vi "ThermoV_ControlSweep_2VO_VG2_nomean_160921.vi"() -> ()   [LabVIEW 2013]
panel:
  out "time/(60*13) indicator":dbl
  out "VGate Mod10 indicator":dbl
  in  "Operate HVpp\nOutput Timer":bool caption="Reset"
  out "modular 13":dbl
  in  "Number of seconds for \neach HVpp case state":dbl=30.0
  out "Elapsed Time (s)":dbl
  out "DC Value":dbl[](array[numeric]) format="%#.6f"
  in  "Saving Avg?":bool
  in  "Filename":path=path "trial_1.lvm"
  in  "STOP":bool
  in  "Save Waveform":bool
  out "Peak2Peak V":dbl[](array[numeric])
  out "Waveform Chart":dynamicdata(graph)
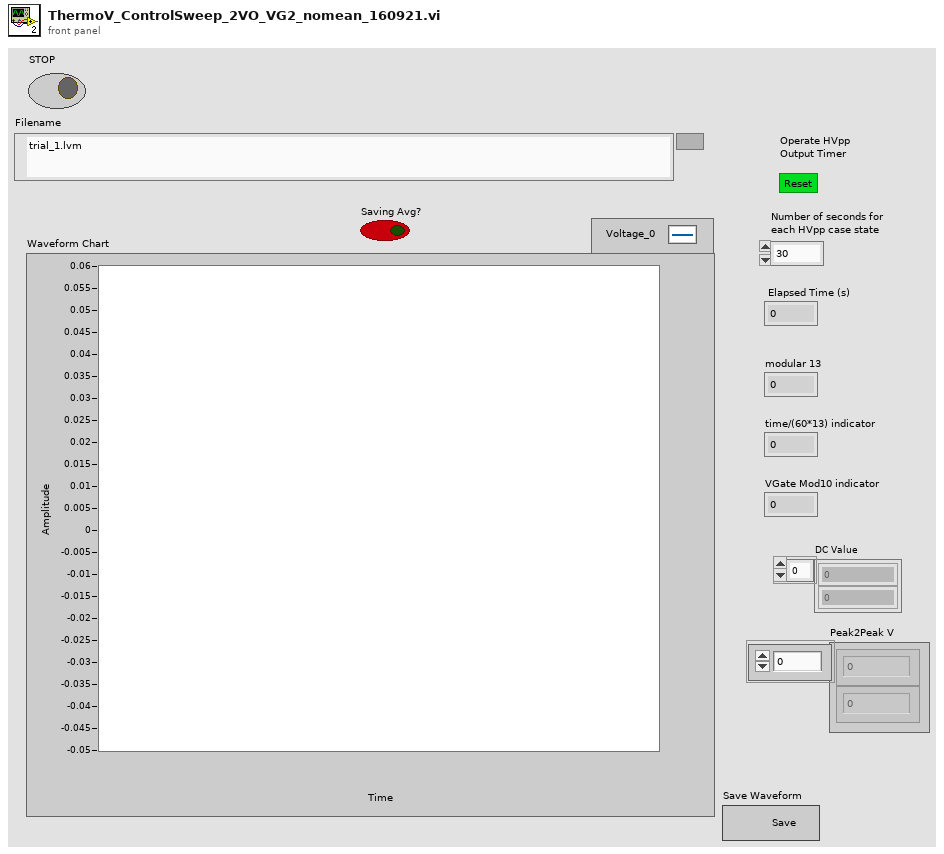
[diagram p1: front panel]
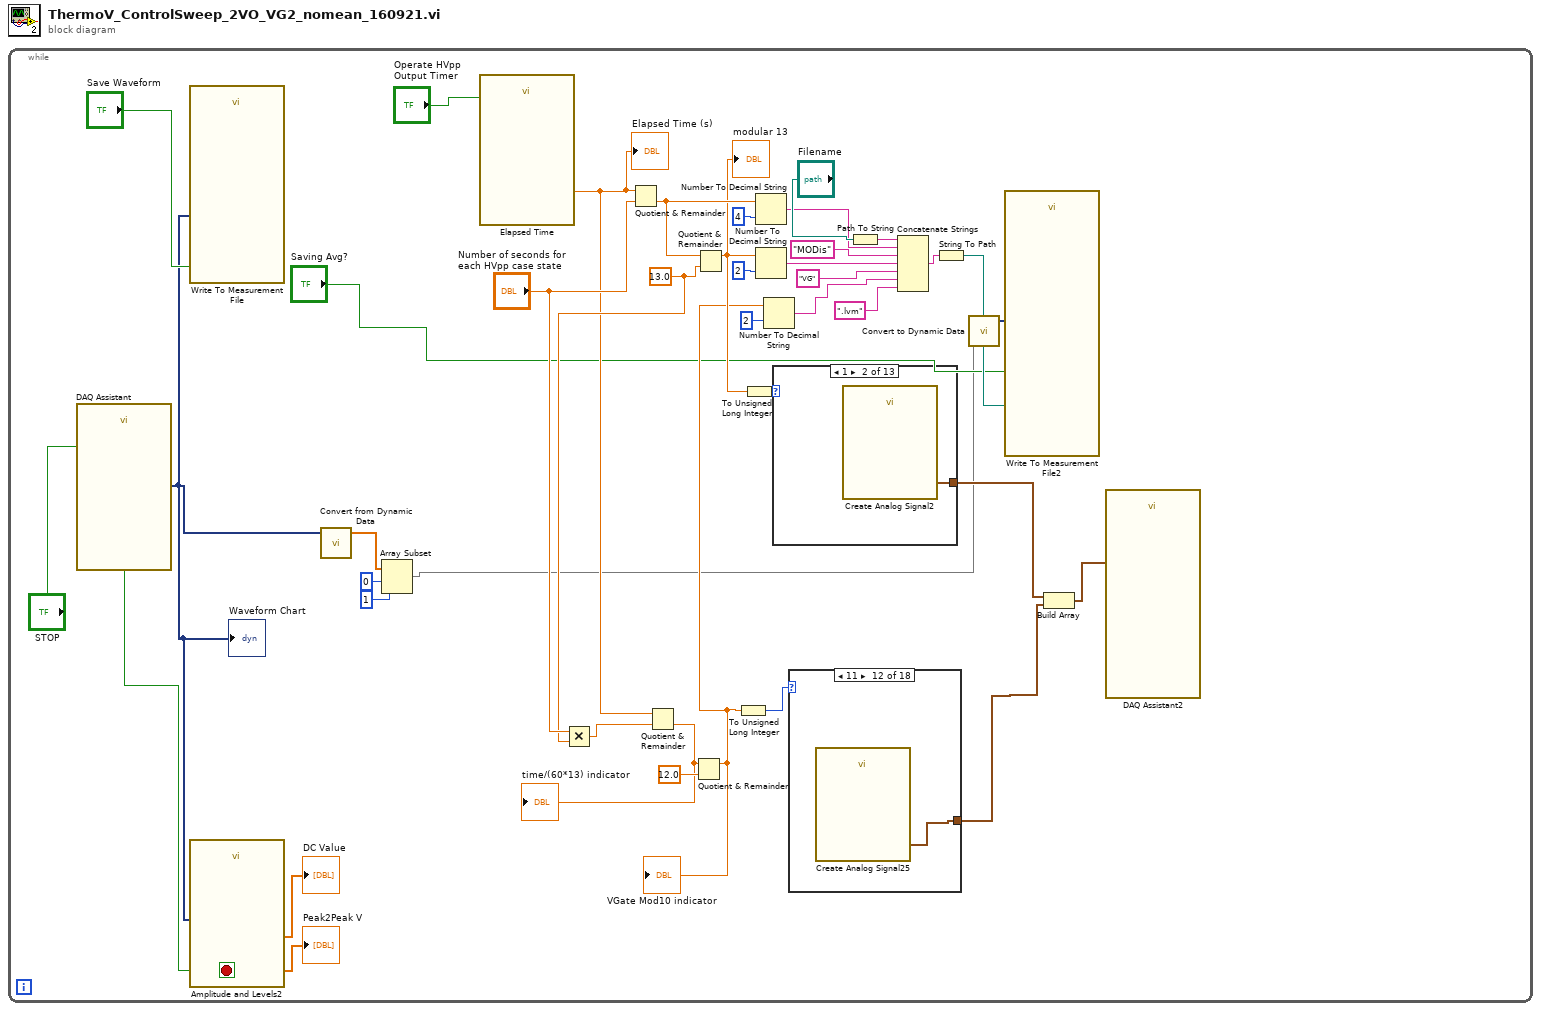
[diagram p0: block diagram]
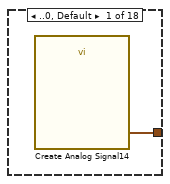
[diagram p2: hidden frame]
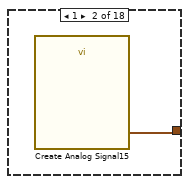
[diagram p3: hidden frame]
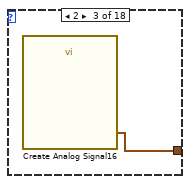
[diagram p4: hidden frame]
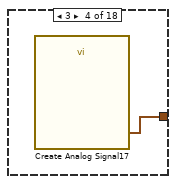
[diagram p5: hidden frame]
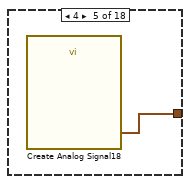
[diagram p6: hidden frame]
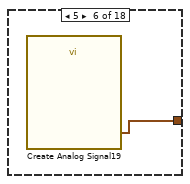
[diagram p7: hidden frame]
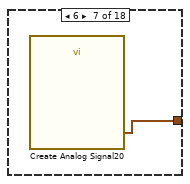
[diagram p8: hidden frame]
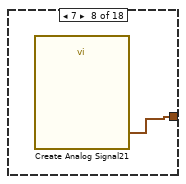
[diagram p9: hidden frame]
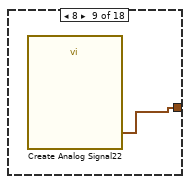
[diagram p10: hidden frame]
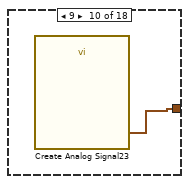
[diagram p11: hidden frame]
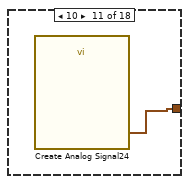
[diagram p12: hidden frame]
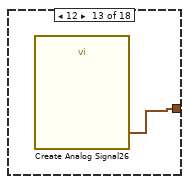
[diagram p13: hidden frame]
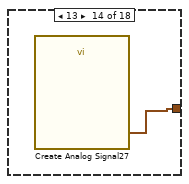
[diagram p14: hidden frame]
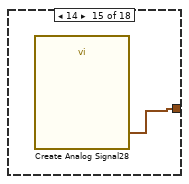
[diagram p15: hidden frame]
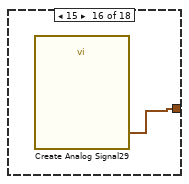
[diagram p16: hidden frame]
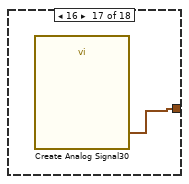
[diagram p17: hidden frame]
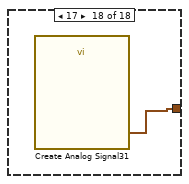
[diagram p18: hidden frame]
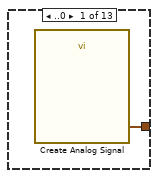
[diagram p19: hidden frame]
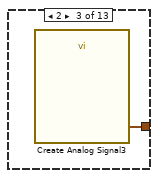
[diagram p20: hidden frame]
diagram:
  n1 = while {
    stop <- w40 stop-if-true
    w20 = 13.0 ("y")
    n2 = call "DAQ Assistant"("stop (F)"="STOP") -> ("data"=w6:dynamicdata, "stopped"=w40:bool)  [unwired: 15 in, 2 out]
    "Waveform Chart" <- w6
    n3 = call "Write To Measurement File"("Signals"=w6, "Enable"="Save Waveform") -> ()  [unwired: 15 in, 3 out]
    n4 = call "Amplitude and Levels2"("input signals"=w6) -> ("dc"=→"DC Value":dbl[], "peak-peak"=→"Peak2Peak V":dbl[])  [unwired: 15 in, 2 out]
    n5 = call "Convert from Dynamic Data"("Dynamic Data Type"=w6) -> ("Array"=w2:dbl[])  [unwired: 3 in]
    n6 = Array Subset(array=w2, index=0, length=1) -> (w3:dbl[])
    n7 = call "Elapsed Time"("Reset"="Operate HVpp\nOutput Timer") -> ("Elapsed Time (s)"=w19:dbl)  [unwired: 11 in, 7 out]
    "Elapsed Time (s)" <- w19
    n8 = Multiply(x="Number of seconds for \neach HVpp case state", y=w20) -> (x*y=w22:dbl)
    n9 = Quotient & Remainder(x=w19, y="Number of seconds for \neach HVpp case state") -> (floor(x/y)=w29:dbl)  [unwired: 1 out]
    n10 = Quotient & Remainder(x=w19, y=w22) -> (floor(x/y)=w13:dbl)  [unwired: 1 out]
    "time/(60*13) indicator" <- w13
    n11 = Quotient & Remainder(x=w13, y=12.0) -> (x-y*floor(x/y)=w12:dbl)  [unwired: 1 out]
    "VGate Mod10 indicator" <- w12
    n12 = Quotient & Remainder(x=w29, y=w20) -> (x-y*floor(x/y)=w25:dbl)  [unwired: 1 out]
    "modular 13" <- w25
    n13 = To Unsigned Long Integer(number=w12) -> (unsigned 32bit integer=w18:u32)
    n14 = To Unsigned Long Integer(number=w25) -> (unsigned 32bit integer=w35:u32)
    n15 = Number To Decimal String(number=w29, width (-)=i16 4) -> (decimal integer string=w28:string)
    n16 = Number To Decimal String(number=w25, width (-)=i16 2) -> (decimal integer string=w24:string)
    n17 = Number To Decimal String(number=w12, width (-)=i16 2) -> (decimal integer string=w15:string)
    n18 = case shown="1" w35 {
      tunnel: [w59 w60 w61 w62 w63 w64 w65 w66 w67 w68 w69 w70 w71] -> w11
      frame ..0 {
        n19 = call "Create Analog Signal"() -> ("sine wave"=w59:waveform(dbl))  [unwired: 18 in, 1 out]
      }
      frame 1 {
        n20 = call "Create Analog Signal2"() -> ("sine wave"=w60:waveform(dbl))  [unwired: 18 in, 1 out]
      }
      frame 2 {
        n21 = call "Create Analog Signal3"() -> ("sine wave"=w61:waveform(dbl))  [unwired: 18 in, 1 out]
      }
      frame 3 {
        n22 = call "Create Analog Signal4"() -> ("sine wave"=w62:waveform(dbl))  [unwired: 18 in, 1 out]
      }
      frame 4 {
        n23 = call "Create Analog Signal5"() -> ("sine wave"=w63:waveform(dbl))  [unwired: 18 in, 1 out]
      }
      frame 5 {
        n24 = call "Create Analog Signal6"() -> ("sine wave"=w64:waveform(dbl))  [unwired: 18 in, 1 out]
      }
      frame 6 {
        n25 = call "Create Analog Signal7"() -> ("sine wave"=w65:waveform(dbl))  [unwired: 18 in, 1 out]
      }
      frame 7 {
        n26 = call "Create Analog Signal8"() -> ("sine wave"=w66:waveform(dbl))  [unwired: 18 in, 1 out]
      }
      frame 8 {
        n27 = call "Create Analog Signal9"() -> ("sine wave"=w67:waveform(dbl))  [unwired: 18 in, 1 out]
      }
      frame 9 {
        n28 = call "Create Analog Signal10"() -> ("sine wave"=w68:waveform(dbl))  [unwired: 18 in, 1 out]
      }
      frame 10 {
        n29 = call "Create Analog Signal11"() -> ("sine wave"=w69:waveform(dbl))  [unwired: 18 in, 1 out]
      }
      frame 11 {
        n30 = call "Create Analog Signal12"() -> ("sine wave"=w70:waveform(dbl))  [unwired: 18 in, 1 out]
      }
      frame 12.. {
        n31 = call "Create Analog Signal13"() -> ("sine wave"=w71:waveform(dbl))  [unwired: 18 in, 1 out]
      }
    }
    n32 = case shown="11" w18 {
      tunnel: [w41 w42 w43 w44 w45 w46 w47 w48 w49 w50 w51 w52 w53 w54 w55 w56 w57 w58] -> w10
      frame ..0, Default {
        n33 = call "Create Analog Signal14"() -> ("DC signal"=w41:waveform(dbl))  [unwired: 18 in, 1 out]
      }
      frame 1 {
        n34 = call "Create Analog Signal15"() -> ("DC signal"=w42:waveform(dbl))  [unwired: 18 in, 1 out]
      }
      frame 2 {
        n35 = call "Create Analog Signal16"() -> ("DC signal"=w43:waveform(dbl))  [unwired: 18 in, 1 out]
      }
      frame 3 {
        n36 = call "Create Analog Signal17"() -> ("DC signal"=w44:waveform(dbl))  [unwired: 18 in, 1 out]
      }
      frame 4 {
        n37 = call "Create Analog Signal18"() -> ("DC signal"=w45:waveform(dbl))  [unwired: 18 in, 1 out]
      }
      frame 5 {
        n38 = call "Create Analog Signal19"() -> ("DC signal"=w46:waveform(dbl))  [unwired: 18 in, 1 out]
      }
      frame 6 {
        n39 = call "Create Analog Signal20"() -> ("DC signal"=w47:waveform(dbl))  [unwired: 18 in, 1 out]
      }
      frame 7 {
        n40 = call "Create Analog Signal21"() -> ("DC signal"=w48:waveform(dbl))  [unwired: 18 in, 1 out]
      }
      frame 8 {
        n41 = call "Create Analog Signal22"() -> ("DC signal"=w49:waveform(dbl))  [unwired: 18 in, 1 out]
      }
      frame 9 {
        n42 = call "Create Analog Signal23"() -> ("DC signal"=w50:waveform(dbl))  [unwired: 18 in, 1 out]
      }
      frame 10 {
        n43 = call "Create Analog Signal24"() -> ("DC signal"=w51:waveform(dbl))  [unwired: 18 in, 1 out]
      }
      frame 11 {
        n44 = call "Create Analog Signal25"() -> ("DC signal"=w52:waveform(dbl))  [unwired: 18 in, 1 out]
      }
      frame 12 {
        n45 = call "Create Analog Signal26"() -> ("DC signal"=w53:waveform(dbl))  [unwired: 18 in, 1 out]
      }
      frame 13 {
        n46 = call "Create Analog Signal27"() -> ("DC signal"=w54:waveform(dbl))  [unwired: 18 in, 1 out]
      }
      frame 14 {
        n47 = call "Create Analog Signal28"() -> ("DC signal"=w55:waveform(dbl))  [unwired: 18 in, 1 out]
      }
      frame 15 {
        n48 = call "Create Analog Signal29"() -> ("DC signal"=w56:waveform(dbl))  [unwired: 18 in, 1 out]
      }
      frame 16 {
        n49 = call "Create Analog Signal30"() -> ("DC signal"=w57:waveform(dbl))  [unwired: 18 in, 1 out]
      }
      frame 17 {
        n50 = call "Create Analog Signal31"() -> ("DC signal"=w58:waveform(dbl))  [unwired: 18 in, 1 out]
      }
    }
    n51 = Path To String(path="Filename") -> (string=w31:string)
    n52 = Concatenate Strings(w31, w28, "MODis" ("string"), w24, "VG" ("string"), w15, ".lvm" ("string")) -> (w32:string)
    n53 = String To Path(string=w32) -> (path=w33:path)
    n54 = call "Convert to Dynamic Data"("Array"=w3) -> ("Dynamic Data Type"=w1:dynamicdata)  [unwired: 3 in]
    n55 = call "Write To Measurement File2"("Signals"=w1, "Enable"="Saving Avg?", "Filename"=w33) -> ()  [unwired: 14 in, 3 out]
    n56 = Build Array(w11, w10) -> (w9:waveform(dbl)[])
    n57 = call "DAQ Assistant2"("data"=w9) -> ()  [unwired: 16 in, 3 out]
  }
